vi "Lim_FileGetImageData.vi"(8 "error in (no error)":errorcluster, 9 "frameindex":i32, 10 "LIMPICTURE in":T3, 11 "hFile in":T2) -> (0 "error out":errorcluster, 1 "LIMLOCALMETADATA":T1 {"dTimeMSec" format="%.2f"}, 2 "LIMPICTURE out":T3, 3 "hFile out":T2)   [LabVIEW 2014, in "ND2_Reader_32.lvlib"]
uses:
  ND2_Reader_32.lvlib
  controls/cluster_LIMPICTURE.ctl
  controls/numeric_LIMFILEHANDLE.ctl
  controls/numeric_LIMRESULT.ctl
  controls/cluster_LIMLOCALMETADATA.ctl
  nd2 reader/SDK/bin/x86/v6_w32_nd2ReadSDK.dll
panel:
  out "LIMRESULT":T4 items=["LIM_OK"=0, "LIM_ERR_UNEXPECTED"=-1, "LIM_ERR_NOTIMPL"=-2, "LIM_ERR_OUTOFMEMORY"=-3, "LIM_ERR_INVALIDARG "=-4, "LIM_ERR_NOINTERFACE"=-5, "LIM_ERR_POINTER"=-6, "LIM_ERR_FAIL"=-9, "LIM_ERR_NOTFOUND"=-13]
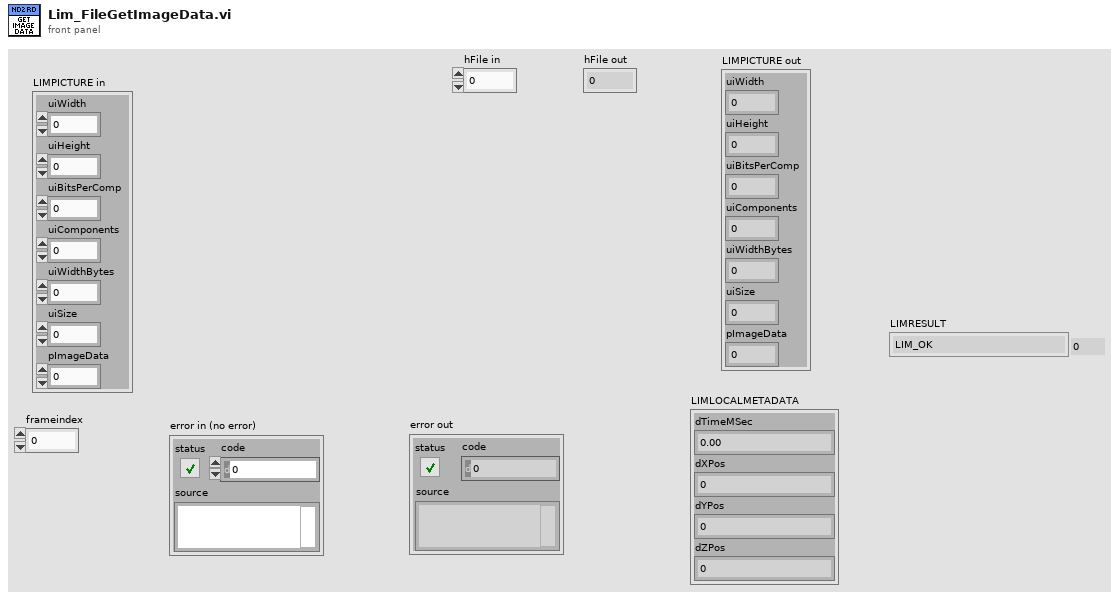
[diagram p1: front panel]
types:
  T1 = typedef "cluster_LIMLOCALMETADATA.ctl" = cluster{"dTimeMSec":dbl, "dXPos":dbl, "dYPos":dbl, "dZPos":dbl}
  T2 = typedef "numeric_LIMFILEHANDLE.ctl" = i32
  T3 = typedef "cluster_LIMPICTURE.ctl" = cluster{"uiWidth":u32, "uiHeight":u32, "uiBitsPerComp":u32, "uiComponents":u32, "uiWidthBytes":u32, "uiSize":u32, "pImageData":u32}
  T4 = typedef "numeric_LIMRESULT.ctl" = i32
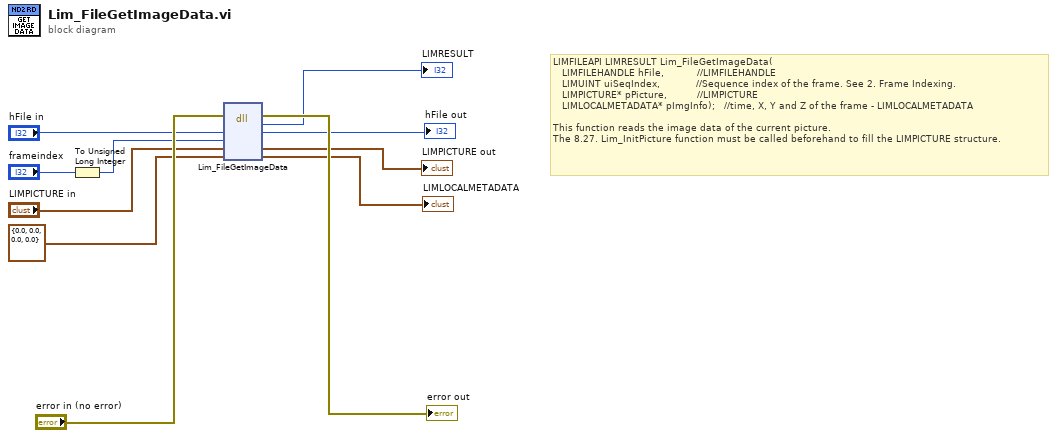
[diagram p0: block diagram]
diagram:
  # "LIMFILEAPI LIMRESULT Lim_FileGetImageData(\n   LIMFILEHANDLE hFile,           //LIMFILEHANDLE \n   LIMUINT uiSeqIndex,            //Sequence index of the frame. See 2. Frame Indexing.\n   LIMPICTURE* pPicture,          //LIMPICTURE\n   LIMLOCALMETADATA* pImgInfo);   //time, X, Y and Z of the frame - LIMLOCALMETADATA\n         \nThis function reads the image data of the current picture. \nThe 8.27. Lim_InitPicture function must be called beforehand to fill the LIMPICTURE structure."
  n1 = To Unsigned Long Integer(number="frameindex") -> (unsigned 32bit integer=w1:u32)
  n2 = dll-call lib="C:/Users/VirtualUser/Desktop/EPA-Vision/EPA Image Source LV2014 2.0.0 2016-02-23/ND2_Reader_32bit/nd2 reader/SDK/bin/x86/v6_w32_nd2ReadSDK.dll" fn="Lim_FileGetImageData"(error in="error in (no error)", "hFile"="hFile in", "uiSeqIndex"=w1, "pPicture"="LIMPICTURE in", "pImgInfo"=T1 {"dTimeMSec"=0.0, "dXPos"=0.0, "dYPos"=0.0, "dZPos"=0.0} ("LIMLOCALMETADATA")) -> (error out=→"error out":errorcluster, "LIMRESULT"=→"LIMRESULT":i32, "hFile"=→"hFile out":i32, "pPicture"=→"LIMPICTURE out":T3, "pImgInfo"=→"LIMLOCALMETADATA":T1)  [unwired: 2 in, 2 out]
